vi "Search DVRs for CSV Path.vi"(8 "error in (no error)":errorcluster, 10 "DVRs":T1[](array[typedef]), 11 "CsvPath":path) -> (0 "error out":errorcluster, 1 "Idx":i32, 2 "Found?":bool, 3 "DVRs dup":T1[](array[typedef]))   [LabVIEW 2011]
uses:
  Controls/DVR of CSV Tests Data.ctl
  Controls/CSVs Tests Data.ctl
  Controls/Test Column Data.ctl
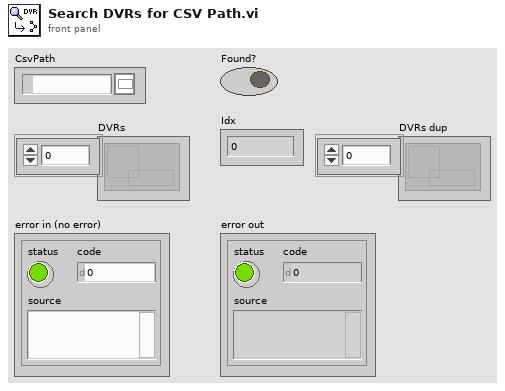
[diagram p1: front panel]
types:
  T1 = typedef "DVR of CSV Tests Data.ctl" = refnum<data-value>
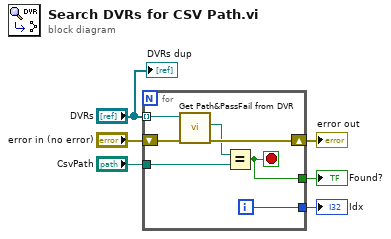
[diagram p0: block diagram]
diagram:
  n1 = for {
    shift-right: [w11] -> w5
    shift-left: "error in (no error)" -> [w13]
    tunnel: "DVRs" -> [w12] mode=indexing
    tunnel: "CsvPath" -> [w10]
    tunnel: [w8] -> w6
    tunnel: [w7] -> w4
    i -> [w8]
    stop <- w7 stop-if-true
    n2 = call "Get Path&PassFail from DVR.vi"("error in (no error)"=w13, "Data Value Reference in"=w12) -> ("error out"=w11:errorcluster, "CsvPath"=w9:path)  [unwired: 5 in, 3 out]
    n3 = Equal?(x=w9, y=w10) -> (x = y?=w7:bool)
  }
  "Idx" <- w6
  "error out" <- w5
  "Found?" <- w4
  "DVRs dup" <- "DVRs"
